vi "Stufen abfragen Tabelle vorbereiten.vi"(8 "Fehler (Eingang)":errorcluster caption="Fehler (Ausgang)", 9 "2D String-Array zum Übersetzen":string[][](array[string]), 10 "Komponente in":u16, 11 "Tabelle (Eingang)":refnum<vi>) -> (0 "Fehler (Ausgang)":errorcluster, 2 "Komponente out":u16, 3 "Tabelle (Ausgang)":refnum<vi>)   [LabVIEW 2020, in "Linearisierung v2.lvlib" / "SpanEinstellungen.lvlib"]
uses:
  SpanEinstellungen.lvlib
  Aktion Lin Daten aufarbeiten.ctl
  Linearisierung v2.lvlib
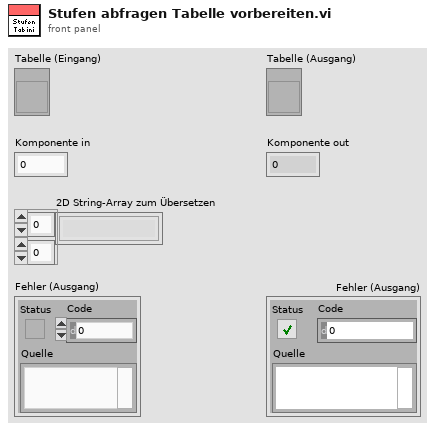
[diagram p1: front panel]
types:
  T1 = typedef "Linearisierung v2.lvlib/Aktion Lin Daten aufarbeiten.ctl" = enum16{"lesen", "Protkolldaten", "speichern", "laden", "EPA auswerten", "Tabelle schreiben", "Lin auswerten", "Tab init", "Stufentabelle", "EPA aktiviert", "Nachbehandlung laden", "Tabelle löschen", "Istwerte löschen", "Zeile löschen", "Zeile einfügen", "LIN aktiviert", "LIN/EPA aktiv laden", "EGAK Tab", "LIN übernehmen", "Tab init ohne Stufen"}
  T2 = typedef "Linearisierung v2.lvlib/Gasteiler.lvlib/Stufen Tabelle.ctl" = string[][]
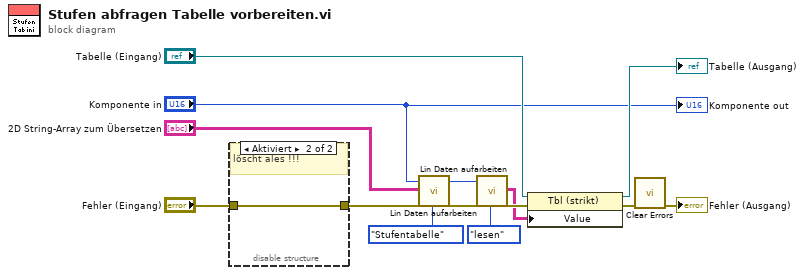
[diagram p0: block diagram]
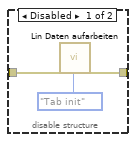
[diagram p2: hidden frame]
diagram:
  n1 = disable-structure shown="Aktiviert" {
    disable-tunnel: [w17 w18] -> w8
    disable-tunnel: "Fehler (Eingang)" -> [w15 w18]
    frame Disabled {
      n2 = call "Lin Daten aufarbeiten.vi"("error in (no error)"=w15, "Aktionen"=Aktion_Lin_Daten_aufarbeiten."Tab init") -> ("error out"=w17:errorcluster)  [unwired: 15 in, 10 out]
    }
    frame Enabled {
      # "löscht ales !!!"
    }
  }
  n3 = call "Lin Daten aufarbeiten.vi"("Index (Seite)"="Komponente in", "Stufen Tabelle"="2D String-Array zum Übersetzen", "error in (no error)"=w8, "Aktionen"=Aktion_Lin_Daten_aufarbeiten."Stufentabelle") -> ("Index (Seite) out"=w11:i32, "error out"=w6:errorcluster)  [unwired: 13 in, 9 out]
  n4 = call "Lin Daten aufarbeiten.vi"("Index (Seite)"=w11, "error in (no error)"=w6, "Aktionen"=Aktion_Lin_Daten_aufarbeiten."lesen") -> ("Stufen Tabelle"=w1:T2, "error out"=w13:errorcluster)  [unwired: 14 in, 9 out]
  n5 = property class="Tbl (strikt)"(reference="Tabelle (Eingang)", error in=w13, "Value"=w1) -> (reference out=→"Tabelle (Ausgang)":refnum<vi>, error out=w10:errorcluster)
  n6 = call <vilib>:"Clear Errors.vi"("error in (no error)"=w10) -> ("error out"=→"Fehler (Ausgang)":errorcluster)  [unwired: 5 in, 1 out]
  "Komponente out" <- "Komponente in"
